vi "PID_Mark10.vi"(5 "Error Previous":dbl, 6 "Input":dbl min=-200.0 max=200.0 format="%.2g", 7 "Error Accumulator":dbl, 8 "Setpoint":dbl min=0.0 max=180.0 format="%_4g", 9 "Kp":dbl min=-100.0 max=200.0 format="%.2f", 10 "Kd":dbl min=-100.0 max=200.0 format="%.2f", 11 "Ki":dbl min=0.0 max=200.0 format="%.2f") -> (1 "Error Previous":dbl, 2 "Error Accumulator":dbl, 3 "Drive out":dbl format="%_3f")   [LabVIEW 2015]
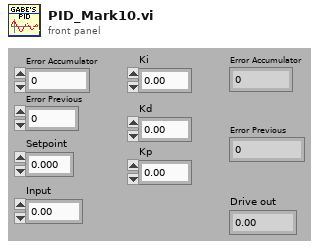
[diagram p1: front panel]
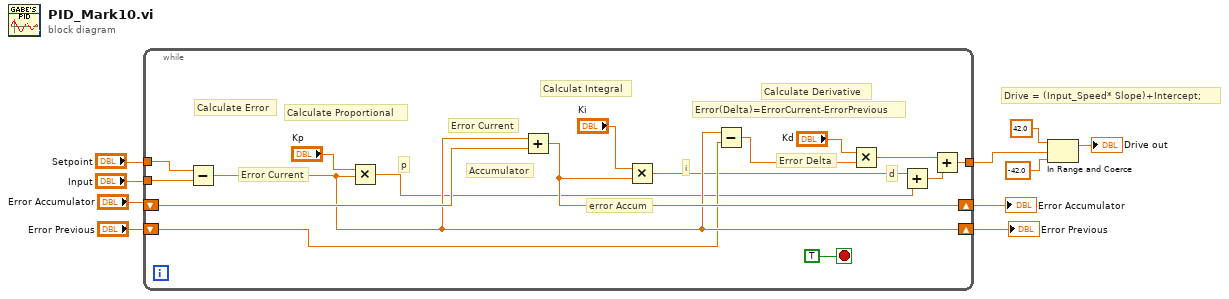
[diagram p0: block diagram]
diagram:
  # "Drive = (Input_Speed* Slope)+Intercept;"
  n1 = while {
    tunnel: "Setpoint" -> [w25]
    tunnel: [w24] -> w7
    tunnel: "Input" -> [w23]
    shift-right: [w16] -> w5
    shift-left: "Error Previous" -> [w15]
    shift-right: [w26] -> w9
    shift-left: "Error Accumulator" -> [w17]
    stop <- TRUE stop-if-true
    # "Error Delta"
    # "d"
    # "Error(Delta)=ErrorCurrent-ErrorPrevious"
    # "Calculate Derivative"
    # "Accumulator"
    # "i"
    # "Error Current"
    # "error Accum"
    # "Calculat Integral"
    # "p"
    # "Calculate Proportional"
    # "Error Current"
    # "Calculate Error"
    n2 = Subtract(x=w25, y=w23) -> (x-y=w16:dbl)
    n3 = Multiply(x="Kp", y=w16) -> (x*y=w14:dbl)
    n4 = Add(x=w16, y=w17) -> (x+y=w26:dbl)
    n5 = Multiply(x="Ki", y=w26) -> (x*y=w13:dbl)
    n6 = Subtract(x=w16, y=w15) -> (x-y=w19:dbl)
    n7 = Multiply(x="Kd", y=w19) -> (x*y=w11:dbl)
    n8 = Add(x=w13, y=w14) -> (x+y=w12:dbl)
    n9 = Add(x=w11, y=w12) -> (x+y=w24:dbl)
  }
  "Error Accumulator" <- w9
  "Error Previous" <- w5
  n10 = In Range and Coerce(upper limit=42.0, x=w7, lower limit=-42.0) -> (coerced(x)=→"Drive out":dbl)  [unwired: 1 out]
